vi "Meas Result Readings Panel.vi"(8 "error in":errorcluster, 11 "meas in":variant) -> (0 "error out":errorcluster, 3 "meas out":variant)   [LabVIEW 2020]
doc: "Panel for manual removal of readings."
uses:
  meas session.ctl
  Meas Sweep Config.ctl
  Meas Freq Info.ctl
  meas_swp_mode.ctl
  meas_sweep_flist_mode.ctl
  bridge/Bridge Session.ctl
  bridge/Bridge Type.ctl
  drivers/TWM client/TWM Session.ctl
  drivers/TWM client/TWM parameters.ctl
  drivers/TWM client/Meas Proc QWTB Uncertainty Mode.ctl
  bridge/Bridge Algorithm.ctl
  bridge/Bridge Bias Session.ctl
  bridge/Bridge Bias Type.ctl
  bridge/Bridge Sim Mode.ctl
  source/Source Session.ctl
  source/Source Type.ctl
  drivers/AFG3101C/AFG3101C Session.ctl
  drivers/cDAQ DDS/cDAQ DDS Session.ctl
  drivers/cDAQ DDS/cDAQ DDS Setup.ctl
  drivers/cDAQ DDS/cDAQ DDS Timebase Mode.ctl
  drivers/cDAQ DDS/cDAQ DDS Dither.ctl
  drivers/Fluke 5XXX/top_lev/F5xxx_session.ctl
  drivers/Fluke 5XXX/top_lev/F5xxx_output_mode.ctl
  Meas Results Ref.ctl
  Meas Results.ctl
  bridge/Bridge Frequency Readings Data.ctl
  drivers/TWM client/Meas Proc QWTB Spectrum Data.ctl
  drivers/TWM client/TWM Phase Info.ctl
  dvm/dvm session.ctl
  dvm/dvm type.ctl
  drivers/Fluke 5790A/top_level/F5790 session.ctl
  thermo/thermo.ctl
  thermo/thermo_types.ctl
  thermo/Thermometer Fail Action.ctl
  Meas Result Major Format.ctl
  varilib/SGUI Assign References Mode.ctl
  Meas Result Formats.ctl
  <vilib>/Utility/miscctls.llb/LVRowAndColumnTypeDef.ctl
  varilib/varilib.lvlib
panel:
  in  "udvm fmt":T1=enum."%_5p" caption="Udvm format"
  in  "udut fmt":T1=enum."%_5p" caption="Udut format"
  in  "iref fmt":T1=enum."%_5p" caption="Iref format"
  in  "table xls":string[][](table) caption="Readings"
  in  "mnr fmt":T1=enum."%_5p" caption="Minor format"
  in  "mjr fmt":T1=enum."%_5p" caption="Major format"
  out "sweep spot index":u16
  out "phase index":u16
  in  "meas in":T2={"swp cfg"={"N"=0, "R"=0, "f list"=[], "smpl delay"=0.0, "set delay"=0.0, "set delay np"=0.0, "meas root"=path "", "meas name"="", "meas a-index"=FALSE, "rnd sweep"=FALSE, "mode"=enum."Frequency", "swp mode"=enum."Linear", "avg"=0, "subrec"=0, "multi-freq"=FALSE, "selfcal"=FALSE, "selfcal period [h]"=0.0}, "bridge"={"type"=enum."TWM client", "TWM"={"pipe name"="", "parameters"=[], "handle"=0, "fixed aper [s]"=0.0, "f-list [Hz]"=[], "discrete f-list"=FALSE, "unc mode"=enum."None", "unc mcc"=0, "unc first"=FALSE, "alg id"=enum."TWM-LowZ - Low Z measurement"}, "last f"=0.0, "bias comp"={"bias type"=enum."dummy", "VISA"="", "Enable"=FALSE, "channel qu"=[], "channel Uinit"=[]}, "sim mode"=enum."Generic RLC network", "channel idns"=[], "sim phases"=1}, "src"={"type"=enum."Tektronix AFG3101C", "afg"={"VISA"="", "const"=0.0, "gen DC"=FALSE, "ext ref"=FALSE}, "cDAQ dds"={"device"="", "channels"=[], "mclk source"="", "mclk [Hz]"=0.0, "fs [Hz]"=0.0, "block [s]"=0.0, "buf [s]"=0.0, "task"="", "cmd queue"=refnum, "proc ref"=refnum, "smpl clock out"="/cDAQ3/PFI0", "export smpl clock"=FALSE, "DC ofs [V]"=[], "timebase source"="", "timebase mode"=enum."Local", "dither"=enum."Disabled", "dither level"=0.0, "phase [rad]"=[]}, "gain [V/A]"=1.0, "F5xxx session"={"VISA"="", "mode"=enum."AC voltage", "Earth on"=FALSE, "Ext ref lock"=FALSE}}, "results"=refnum, "dvm"={"type"=enum."Disabled", "F5790"={"VISA"="", "Input"=enum."input 1", "Digital filter restart"=enum."medium", "hi resolution"=enum."off", "Digital filter mode"=enum."off", "ext guard"=FALSE}}, "thermo"={"type"=enum."COMET Tx5xx (ethernet)", "comment"="", "tag"="", "refresh"=5.0, "IP"="", "port"=502, "VISA"="", "last readout"=timestamp(0 s since 1904-01-01), "TCP ref"=refnum, "VISA sess"="", "idn"="", "press"=0.0, "RH"=0.0, "temp"=0.0, "pres cor"=[], "RH cor"=[], "temp cor"=[], "try left"=0, "failed"=FALSE, "RTD set"=[], "RTD inv"=[], "range"=0.0, "net mode"=enum."MODBUS", "try fail"=enum."Stop trying - return NaN", "timeout [s]"=0.0, "max retries"=0, "sim t [deg]"=0.0}} {"thermo"."RTD inv" format="%.1f"; "thermo"."RTD set" format="%.1f"; "thermo"."temp cor" format="%.1f"; "thermo"."RH cor" format="%.1f"; "thermo"."pres cor" format="%.1f"; "thermo"."refresh" min=0.1 max=1000.0 format="%.2f"; "src"."cDAQ dds"."channels" min=0 step=1; "bridge"."TWM"."f-list [Hz]" format="%#_6p"; "swp cfg"."f list"."bias" format="%#_3p"; "swp cfg"."f list"."level" format="%#_3p"; "swp cfg"."f list"."fs [Hz]" format="%#_5p"; "swp cfg"."f list"."time [s]" format="%#_3p"; "swp cfg"."f list"."f/fs" format="%#_3p"; "swp cfg"."f list"."periods" format="%#_3f"; "swp cfg"."f list"."f [Hz]" format="%#_5p"}
  in  "btn rem":bool
  in  "rdgs ring spot":u16(ring) caption="Sweep spot selection" items=["Last measured", "#1, f=53.00Hz, Iac=1.000A, Idc=0.000A", "#2, f=70.00Hz, Iac=1.000A, Idc=0.000A", "#3, f=97.00Hz, Iac=1.000A, Idc=0.000A", "#4, f=136.0Hz, Iac=1.000A, Idc=0.000A", "#5, f=189.0Hz, Iac=1.000A, Idc=0.000A", "#6, f=264.0Hz, Iac=1.000A, Idc=0.000A", "#7, f=368.0Hz, Iac=1.000A, Idc=0.000A", "#8, f=514.0Hz, Iac=1.000A, Idc=0.000A", "#9, f=717.0Hz, Iac=1.000A, Idc=0.000A", "#10, f=1.000kHz, Iac=1.000A, Idc=0.000A"]
  in  "rdgs ring phase":u16(ring) caption="Phase selection" items=["L1"]
  in  "btn ok":bool
  in  "table":string[][](table) caption="Readings (right click to show actions)"
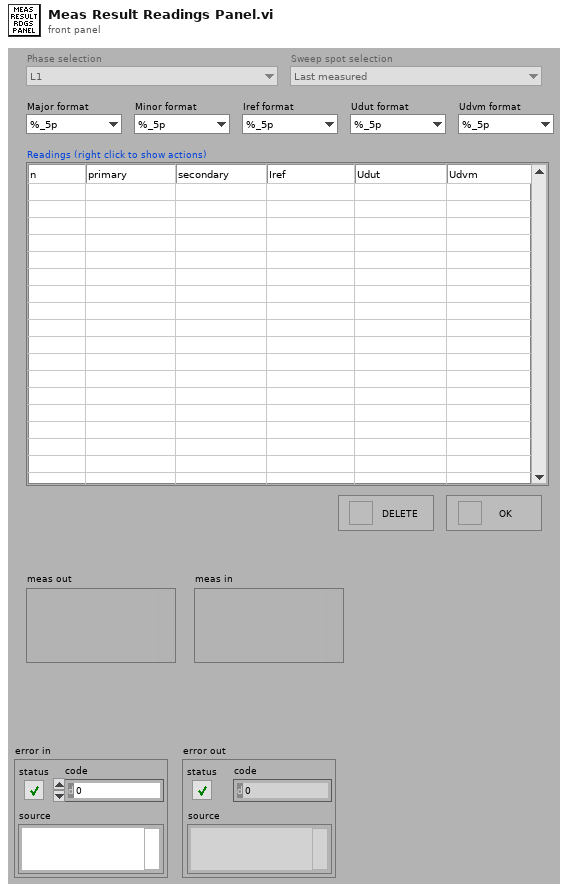
[diagram p1: front panel]
types:
  T1 = typedef "Meas Result Major Format.ctl" = enum16{"%_3p", "%_4p", "%_5p", "%_6p", "%_7p", "%_8p", "%_5f", "%_6f", "%_7f", "%_8f", "%_5e", "%_6e", "%_7e", "%_8e", "%.4f", "%.5f", "%.6f", "%.7f"}
  T2 = typedef "meas session.ctl" = cluster{"swp cfg":T3, "bridge":T7, "src":T16, "results":T24, "dvm":T25, "thermo":T28}
  T3 = typedef "Meas Sweep Config.ctl" = cluster{"N":i32, "R":i32, "f list":T4[], "smpl delay":dbl, "set delay":dbl, "set delay np":dbl, "meas root":path, "meas name":string, "meas a-index":bool, "rnd sweep":bool, "mode":T5, "swp mode":T6, "avg":i32, "subrec":i32, "multi-freq":bool, "selfcal":bool, "selfcal period [h]":dbl}
  T4 = typedef "Meas Freq Info.ctl" = cluster{"f [Hz]":dbl, "periods":dbl, "f/fs":dbl, "time [s]":dbl, "fs [Hz]":dbl, "N":i32, "level":dbl, "bias":dbl, "rdgs":i32, "f. id":i32}
  T5 = typedef "meas_swp_mode.ctl" = enum16{"Frequency", "Level", "Bias"}
  T6 = typedef "meas_sweep_flist_mode.ctl" = enum16{"Linear", "Log10"}
  T7 = typedef "Bridge Session.ctl" = cluster{"type":T8, "TWM":T9, "last f":dbl, "bias comp":T13, "sim mode":T15, "channel idns":string[], "sim phases":i32}
  T8 = typedef "Bridge Type.ctl" = enum16{"TWM client", "dummy"}
  T9 = typedef "TWM Session.ctl" = cluster{"pipe name":string, "parameters":T10[], "handle":i32, "fixed aper [s]":dbl, "f-list [Hz]":dbl[], "discrete f-list":bool, "unc mode":T11, "unc mcc":i32, "unc first":bool, "alg id":T12}
  T10 = typedef "TWM parameters.ctl" = cluster{"name":string, "value":string[]}
  T11 = typedef "Meas Proc QWTB Uncertainty Mode.ctl" = enum16{"None", "GUF", "Monte Carlo"}
  T12 = typedef "Bridge Algorithm.ctl" = enum16{"TWM-LowZ - Low Z measurement", "TWM-InpZ - Digitizer input Z measurement", "TWM-TIAZ - High Z using TIA"}
  T13 = typedef "Bridge Bias Session.ctl" = cluster{"bias type":T14, "VISA":refnum<visa-resource-name>, "Enable":bool, "channel qu":string[], "channel Uinit":dbl[]}
  T14 = typedef "Bridge Bias Type.ctl" = enum16{"dummy", "CMI LiBbias V1.0"}
  T15 = typedef "Bridge Sim Mode.ctl" = enum16{"Generic RLC network", "Interchannel transfer", "Input impedance"}
  T16 = typedef "Source Session.ctl" = cluster{"type":T17, "afg":T18, "cDAQ dds":T19, "gain [V/A]":dbl, "F5xxx session":T22}
  T17 = typedef "Source Type.ctl" = enum16{"Tektronix AFG3101C", "cDAQ DAC", "Fluke 5xxx", "Agilent 33120A", "dummy"}
  T18 = typedef "AFG3101C Session.ctl" = cluster{"VISA":refnum<visa-resource-name>, "const":dbl, "gen DC":bool, "ext ref":bool}
  T19 = typedef "cDAQ DDS Session.ctl" = cluster{"device":tag, "channels":i32[], "mclk source":tag, "mclk [Hz]":dbl, "fs [Hz]":dbl, "block [s]":dbl, "buf [s]":dbl, "task":refnum<k21>, "cmd queue":refnum<queue>, "proc ref":refnum<vi>, "smpl clock out":tag, "export smpl clock":bool, "DC ofs [V]":dbl[], "timebase source":tag, "timebase mode":T20, "dither":T21, "dither level":dbl, "phase [rad]":dbl[]}
  T20 = typedef "cDAQ DDS Timebase Mode.ctl" = enum16{"Local", "Take from ADC (e.g. NI 9238)", "Other source"}
  T21 = typedef "cDAQ DDS Dither.ctl" = enum16{"Disabled", "Gaussian"}
  T22 = typedef "F5xxx_session.ctl" = cluster{"VISA":refnum<visa-resource-name>, "mode":T23, "Earth on":bool, "Ext ref lock":bool}
  T23 = typedef "F5xxx_output_mode.ctl" = enum16{"AC voltage", "AC current"}
  T24 = typedef "Meas Results Ref.ctl" = refnum<vi>
  T25 = typedef "dvm session.ctl" = cluster{"type":T26, "F5790":T27}
  T26 = typedef "dvm type.ctl" = enum16{"Disabled", "Simulated", "Fluke 5790A"}
  T27 = typedef "F5790 session.ctl" = cluster{"VISA":refnum<visa-resource-name>, "Input":enum16{"input 1", "input 2", "wide-band"}, "Digital filter restart":enum16{"medium", "fine", "coarse"}, "hi resolution":enum16{"off", "on"}, "Digital filter mode":enum16{"off", "fast", "medium", "slow"}, "ext guard":bool}
  T28 = typedef "thermo.ctl" = cluster{"type":T29, "comment":string, "tag":string, "refresh":dbl, "IP":string, "port":u16, "VISA":refnum<visa-resource-name>, "last readout":timestamp, "TCP ref":refnum<k5>, "VISA sess":refnum<visa-resource-name>, "idn":string, "press":dbl, "RH":dbl, "temp":dbl, "pres cor":dbl[][], "RH cor":dbl[][], "temp cor":dbl[][], "try left":i32, "failed":bool, "RTD set":dbl[], "RTD inv":dbl[], "range":dbl, "net mode":enum16{"MODBUS", "HTTP"}, "try fail":T30, "timeout [s]":dbl, "max retries":i32, "sim t [deg]":dbl}
  T29 = typedef "thermo_types.ctl" = enum16{"Disabled", "Simulated", "COMET Tx5xx (ethernet)", "Keithley 2002 (GPIB) + RTD", "Agilent 344xx (GPIB) + RTD"}
  T30 = typedef "Thermometer Fail Action.ctl" = enum16{"Stop trying - keep last value", "Stop trying - return NaN", "Generate error - stop sweep"}
  T31 = typedef "varilib.lvlib/SGUI Assign References Mode.ctl" = enum16{"Add to stack", "Overwrite", "Release last", "Release ID"}
  T32 = typedef "Meas Result Formats.ctl" = cluster{"mjr fmt":T1, "mnr fmt":T1, "iref fmt":T1, "udut fmt":T1, "udvm fmt":T1}
  T33 = typedef "LVRowAndColumnTypeDef.ctl" = cluster{"Row":i32, "Column":i32}
  T34 = typedef "Meas Results.ctl" = cluster{"freqs":T35[][], "locked":bool, "last fid":i32, "modified":bool, "mjr name":string, "mnr name":string, "last spectra":T36[][], "saved?":bool, "TWM phase":T37[], "time start":timestamp, "time stop":timestamp, "equ cct":string}
  T35 = typedef "Bridge Frequency Readings Data.ctl" = cluster{"Udut":dbl[], "Iref":dbl[], "Udc":dbl[], "Idc":dbl[], "mjr":dbl[], "mnr":dbl[], "mjr_sh":dbl[], "mnr_sh":dbl[], "u(mjr)":dbl[], "u(mnr)":dbl[], "ua2(mjr)":dbl[], "ua2(mnr)":dbl[], "n":i32, "f [Hz]":dbl, "fs [Hz]":dbl, "aperture [s]":dbl, "Udvm":dbl[], "u(Udvm) [V]":dbl, "t_dut [degC]":dbl[], "RH_dut [%]":dbl[], "p_dut [Pa]":dbl[]}
  T36 = typedef "Meas Proc QWTB Spectrum Data.ctl" = cluster{"x":sgl[], "y":sgl[], "label":string}
  T37 = typedef "TWM Phase Info.ctl" = cluster{"ref chn id (I)":string, "dut chn id (U)":string, "ref chn range [V]":dbl, "dut chn range [V]":dbl, "aperture [s]":dbl, "fs [Hz]":dbl, "ref chn transducer (I)":string, "dut chn transducer (U)":string}
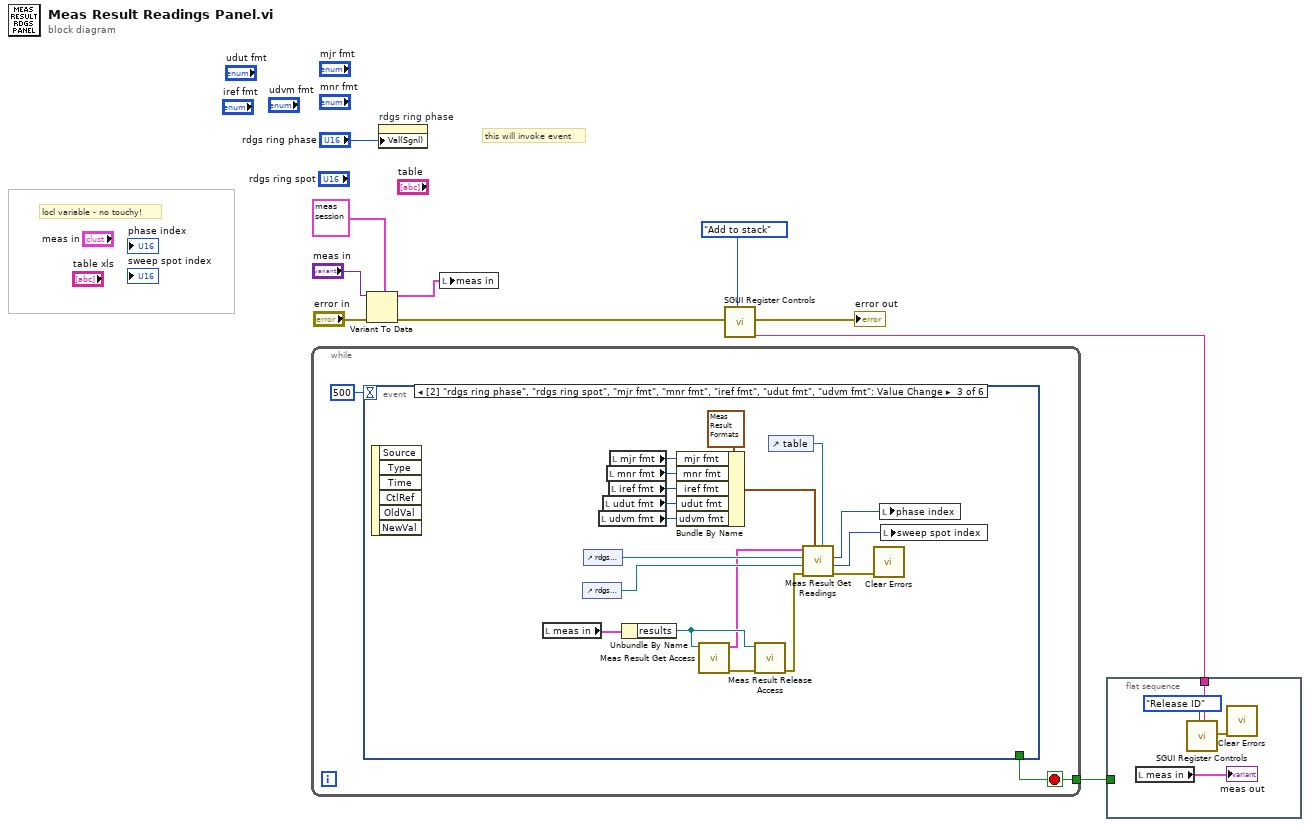
[diagram p0: block diagram]
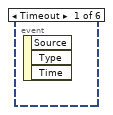
[diagram p2: hidden frame]
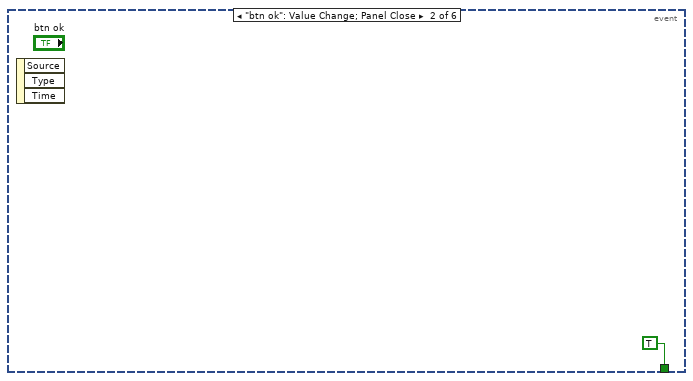
[diagram p3: hidden frame]
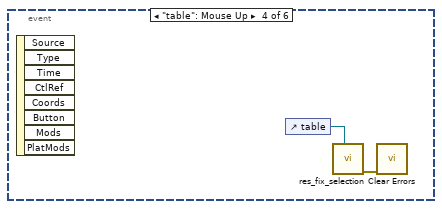
[diagram p4: hidden frame]
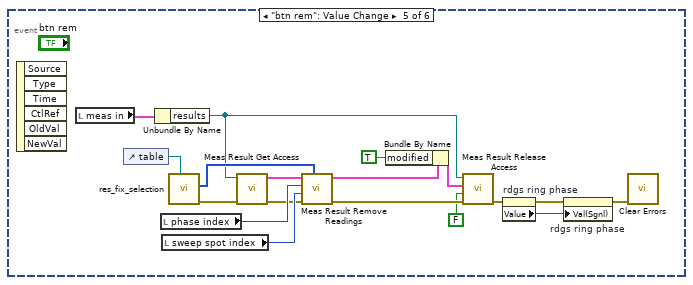
[diagram p5: hidden frame]
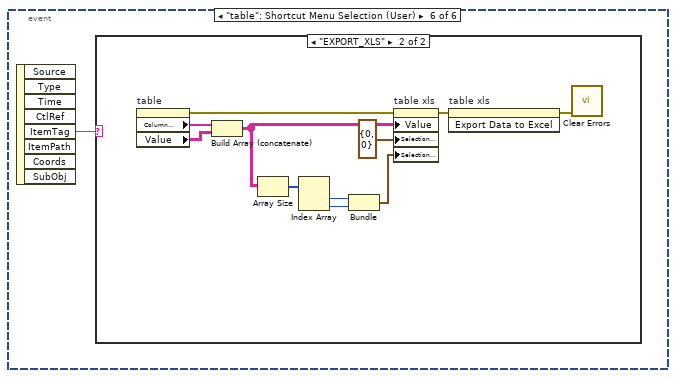
[diagram p6: hidden frame]
diagram:
  # "locl variable - no touchy!"
  # "this will invoke event"
  n1 = while {
    tunnel: [w12] -> w5
    stop <- w12 stop-if-true
    n2 = event shown="[2] \"rdgs ring phase\", \"rdgs ring spot\", \"mjr fmt\", \"mnr fmt\", \"iref fmt\", \"udut fmt\", \"udvm fmt\": Value Change" {
      selector: _ -> [_ _ _ _ _ _]
      dyn-events: _ -> [_ _ _ _ _ _]
      timeout: 500 -> [_ _ _ _ _ _]
      tunnel: [_ TRUE _ _ _ _] -> w12
      event Timeout {
        n3 = event-data() -> ()  [unwired: 1 in, 3 out]
      }
      event "btn ok": Value Change; Panel Close {
        n4 = event-data() -> ()  [unwired: 1 in, 3 out]
      }
      event "rdgs ring phase", "rdgs ring spot": Value Change {
        n5 = event-data() -> ()  [unwired: 1 in, 6 out]
        n6 = local read "meas in"() -> (w27:T2)
        n7 = control-ref of="rdgs ring spot"() -> (w30:refnum<vi>)
        n8 = control-ref of="rdgs ring phase"() -> (w31:refnum<vi>)
        n9 = local read "udvm fmt"() -> (w15:T1)
        n10 = local read "udut fmt"() -> (w16:T1)
        n11 = local read "mnr fmt"() -> (w18:T1)
        n12 = local read "iref fmt"() -> (w17:T1)
        n13 = local read "mjr fmt"() -> (w19:T1)
        n14 = Unbundle By Name(w27) -> ("results"=w28:T24)
        n15 = Bundle By Name(cluster=T32 {"mjr fmt"=enum."%_5p", "mnr fmt"=enum."%_5p", "iref fmt"=enum."%_5p", "udut fmt"=enum."%_5p", "udvm fmt"=enum."%_5p"} ("formats"), "mjr fmt"=w19, "mnr fmt"=w18, "iref fmt"=w17, "udut fmt"=w16, "udvm fmt"=w15) -> (w14:T32)
        n16 = call "Meas Result Get Access.vi"("results ref"=w28) -> ("error out"=w29:errorcluster, "results data"=w26:T34)  [unwired: 9 in]
        n17 = call "Meas Result Release Access.vi"("error in"=w29, "results ref"=w28) -> ("error out"=w24:errorcluster)  [unwired: 9 in]
        n18 = control-ref of="table"() -> (w25:refnum<vi>)
        n19 = call "Meas Result Get Readings.vi"("table ref"=w25, "formats"=w14, "error in (no error)"=w24, "ring spot"=w30, "ring phase"=w31, "result"=w26) -> ("error out"=w23:errorcluster, "sweep spot index"=w21:u16, "phase index"=w22:u16)  [unwired: 1 in, 2 out]
        n20 = call <vilib>:"Clear Errors.vi"("error in (no error)"=w23) -> ()  [unwired: 5 in, 2 out]
        n21 = local write "phase index"(w22) -> ()
        n22 = local write "sweep spot index"(w21) -> ()
      }
      event "table": Mouse Up {
        n23 = event-data() -> ()  [unwired: 1 in, 8 out]
        n24 = control-ref of="table"() -> (w33:refnum<vi>)
        n25 = call "res_fix_selection.vi"("list"=w33) -> ("error out"=w32:errorcluster)  [unwired: 8 in, 2 out]
        n26 = call <vilib>:"Clear Errors.vi"("error in (no error)"=w32) -> ()  [unwired: 5 in, 2 out]
      }
      event "btn rem": Value Change {
        n27 = event-data() -> ()  [unwired: 1 in, 6 out]
        n28 = local read "meas in"() -> (w44:T2)
        n29 = control-ref of="table"() -> (w45:refnum<vi>)
        n30 = Unbundle By Name(w44) -> ("results"=w42:T24)
        n31 = local read "phase index"() -> (w51:u16)
        n32 = local read "sweep spot index"() -> (w50:u16)
        n33 = call "res_fix_selection.vi"("list"=w45) -> ("error out"=w49:errorcluster, "ids of selected"=w43:i32[])  [unwired: 8 in, 1 out]
        n34 = call "Meas Result Get Access.vi"("error in"=w49, "results ref"=w42) -> ("error out"=w48:errorcluster, "results data"=w47:T34)  [unwired: 8 in]
        n35 = call "Meas Result Remove Readings.vi"("ids of selected"=w43, "error in"=w48, "sweep spot index"=w50, "phase index"=w51, "result"=w47) -> ("error out"=w46:errorcluster, "result out"=w36:T34)  [unwired: 5 in]
        n36 = Bundle By Name(cluster=w36, "modified"=TRUE) -> (w35:T34)
        n37 = call "Meas Result Release Access.vi"("error in"=w46, "Release only (True)"=FALSE, "results data in"=w35, "results ref"=w42) -> ("error out"=w40:errorcluster)  [unwired: 7 in]
        n38 = property on="rdgs ring phase" class="Ring (strict)"(error in=w40) -> (error out=w38:errorcluster, "Value"=w39:u16)  [unwired: 1 in, 1 out]
        n39 = property on="rdgs ring phase" class="Ring (strict)"(error in=w38, "Val(Sgnl)"=w39) -> (error out=w37:errorcluster)  [unwired: 1 in, 1 out]
        n40 = call <vilib>:"Clear Errors.vi"("error in (no error)"=w37) -> ()  [unwired: 5 in, 2 out]
      }
      event "table": Shortcut Menu Selection (User) {
        n41 = event-data() -> ("ItemTag"=w52:string)  [unwired: 1 in, 7 out]
        n42 = case shown="\"EXPORT_XLS\"" w52 {
          frame "False", Default {
          }
          frame "EXPORT_XLS" {
            n43 = property on="table" class="Tbl (strict)"() -> (error out=w60:errorcluster, "Column Headers[]"=w62:string[], "Value"=w61:string[][])  [unwired: 2 in, 1 out]
            n44 = Build Array (concatenate)(w62, w61) -> (w59:string[][])
            n45 = Array Size(array=w59) -> (size(s)=w63:i32[])
            n46 = Index Array(array=w63) -> (element #1=w56:i32, element #2=w57:i32)  [unwired: 2 in]
            n47 = Bundle(w56, w57) -> (w55:cluster{i32, i32})  [unwired: 1 in]
            n48 = property on="table xls" class="Tbl (strict)"(error in=w60, "Value"=w59, "Selection Start"=T33 {"Row"=0, "Column"=0}, "Selection Size"=w55) -> (error out=w54:errorcluster)  [unwired: 1 in, 1 out]
            n49 = invoke on="table xls" class="Tbl (strict)" method="Export Data to Excel"(error in=w54) -> (error out=w53:errorcluster)  [unwired: 2 in, 2 out]
            n50 = call <vilib>:"Clear Errors.vi"("error in (no error)"=w53) -> ()  [unwired: 5 in, 2 out]
          }
        }
      }
    }
  }
  n51 = Variant To Data(error in="error in", type=T2 {"swp cfg"={"N"=0, "R"=0, "f list"=[], "smpl delay"=0.0, "set delay"=0.0, "set delay np"=0.0, "meas root"=path "", "meas name"="", "meas a-index"=FALSE, "rnd sweep"=FALSE, "mode"=enum."Frequency", "swp mode"=enum."Linear", "avg"=0, "subrec"=0, "multi-freq"=FALSE, "selfcal"=FALSE, "selfcal period [h]"=0.0}, "bridge"={"type"=enum."TWM client", "TWM"={"pipe name"="", "parameters"=[], "handle"=0, "fixed aper [s]"=0.0, "f-list [Hz]"=[], "discrete f-list"=FALSE, "unc mode"=enum."None", "unc mcc"=0, "unc first"=FALSE, "alg id"=enum."TWM-LowZ - Low Z measurement"}, "last f"=0.0, "bias comp"={"bias type"=enum."dummy", "VISA"="", "Enable"=FALSE, "channel qu"=[], "channel Uinit"=[]}, "sim mode"=enum."Generic RLC network", "channel idns"=[], "sim phases"=1}, "src"={"type"=enum."Tektronix AFG3101C", "afg"={"VISA"="", "const"=0.0, "gen DC"=FALSE, "ext ref"=FALSE}, "cDAQ dds"={"device"="", "channels"=[], "mclk source"="", "mclk [Hz]"=0.0, "fs [Hz]"=0.0, "block [s]"=0.0, "buf [s]"=0.0, "task"="", "cmd queue"=refnum, "proc ref"=refnum, "smpl clock out"="/cDAQ3/PFI0", "export smpl clock"=FALSE, "DC ofs [V]"=[], "timebase source"="", "timebase mode"=enum."Local", "dither"=enum."Disabled", "dither level"=0.0, "phase [rad]"=[]}, "gain [V/A]"=1.0, "F5xxx session"={"VISA"="", "mode"=enum."AC voltage", "Earth on"=FALSE, "Ext ref lock"=FALSE}}, "results"=refnum, "dvm"={"type"=enum."Disabled", "F5790"={"VISA"="", "Input"=enum."input 1", "Digital filter restart"=enum."medium", "hi resolution"=enum."off", "Digital filter mode"=enum."off", "ext guard"=FALSE}}, "thermo"={"type"=enum."COMET Tx5xx (ethernet)", "comment"="", "tag"="", "refresh"=5.0, "IP"="", "port"=502, "VISA"="", "last readout"=timestamp(0 s since 1904-01-01), "TCP ref"=refnum, "VISA sess"="", "idn"="", "press"=0.0, "RH"=0.0, "temp"=0.0, "pres cor"=[], "RH cor"=[], "temp cor"=[], "try left"=0, "failed"=FALSE, "RTD set"=[], "RTD inv"=[], "range"=0.0, "net mode"=enum."MODBUS", "try fail"=enum."Stop trying - return NaN", "timeout [s]"=0.0, "max retries"=0, "sim t [deg]"=0.0}} ("meas in"), Variant="meas in") -> (data=w6:T2, error out=w1:errorcluster)
  n52 = property on="rdgs ring phase" class="Ring (strict)"("Val(Sgnl)"="rdgs ring phase") -> ()  [unwired: 2 in, 2 out]
  n53 = local write "meas in"(w6) -> ()
  n54 = call "SGUI Register Controls.vi"("error in"=w1, "register mode (overwrite)"=SGUI_Assign_References_Mode."Add to stack") -> ("assigned ID"=w2:string, "error out"=→"error out":errorcluster)  [unwired: 15 in, 1 out]
  n55 = flat-sequence {
    tunnel: w5 -> [_]
    tunnel: w2 -> [w66]
    frame #0 {
      n56 = local read "meas in"() -> (→"meas out":T2)
      n57 = call "SGUI Register Controls.vi"("register mode (overwrite)"=SGUI_Assign_References_Mode."Release ID", "controls ID (empty)"=w66) -> ("error out"=w65:errorcluster)  [unwired: 15 in, 2 out]
      n58 = call <vilib>:"Clear Errors.vi"("error in (no error)"=w65) -> ()  [unwired: 5 in, 2 out]
    }
  }
